vi "handle HTTP Error.vi"(8 "httpResponse":refnum<class "httpResponse.lvclass">, 11 "error in (no error)":errorcluster) -> (0 "httpResponse out":refnum<class "httpResponse.lvclass">, 3 "error out":errorcluster)   [LabVIEW 2020, in "httpClient.lvlib" / "httpClient.lvclass"]
uses:
  httpClient.lvclass
  httpResponse/httpResponse.lvclass
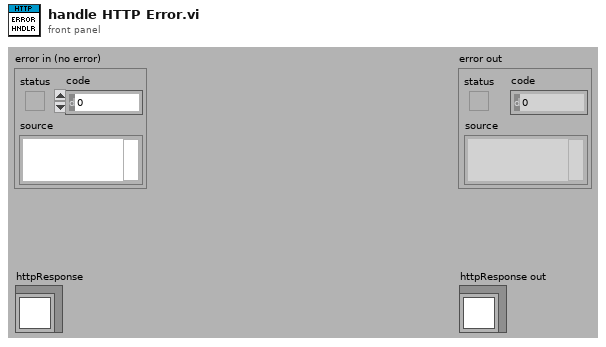
[diagram p1: front panel]
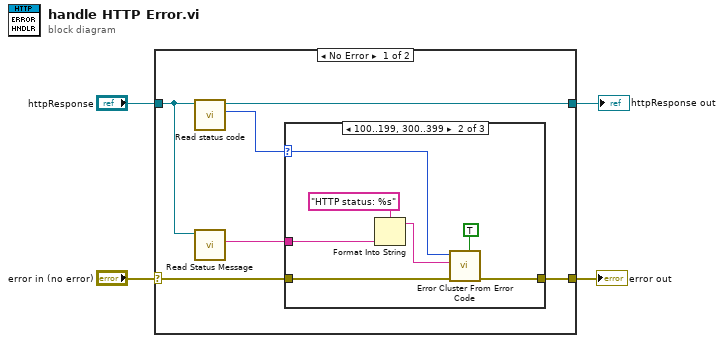
[diagram p0: block diagram]
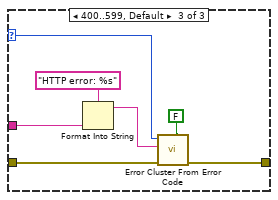
[diagram p3: hidden frame]
diagram:
  n1 = case shown="No Error" "error in (no error)" {
    selector: "error in (no error)" -> [w10 w27]
    tunnel: [w9 w27] -> w3
    tunnel: "httpResponse" -> [w5 w26]
    tunnel: [w6 w26] -> w1
    frame No Error {
      n2 = call "Read status code.vi"("httpResponse in"=w5) -> ("status code"=w8:u16, "httpResponse out"=w6:refnum<class "httpResponse.lvclass">)  [unwired: 9 in]
      n3 = call "Read Status Message.vi"("httpResponse in"=w5) -> ("status message"=w7:string)  [unwired: 9 in, 1 out]
      n4 = case shown="100..199, 300..399" w8 {
        selector: w8 -> [_ w16 w25]
        tunnel: w7 -> [_ w12 w21]
        tunnel: w10 -> [w11 w17 w20]
        tunnel: [w11 w18 w19] -> w9
        frame 200..299 {
          # "Expected response"
        }
        frame 100..199, 300..399 {
          n5 = Format Into String(format string="HTTP status: %s", w12) -> (resulting string=w13:string)  [unwired: 2 in, 1 out]
          n6 = call <vilib>:"Error Cluster From Error Code.vi"("is warning? (False)"=TRUE, "error in (no error)"=w17, "error message (\"\")"=w13, "error code (0)"=w16) -> ("error out"=w18:errorcluster)  [unwired: 5 in]
        }
        frame 400..599, Default {
          n7 = Format Into String(format string="HTTP error: %s", w21) -> (resulting string=w22:string)  [unwired: 2 in, 1 out]
          n8 = call <vilib>:"Error Cluster From Error Code.vi"("is warning? (False)"=FALSE, "error in (no error)"=w20, "error message (\"\")"=w22, "error code (0)"=w25) -> ("error out"=w19:errorcluster)  [unwired: 5 in]
        }
      }
    }
    frame Error {
    }
  }
  "error out" <- w3
  "httpResponse out" <- w1
